vi "SetSendFileProperties.vi"(10 "acqusition timestamp":string, 11 "data group":string) -> (3 "send file properties":T1[](array[typedef]))   [LabVIEW 2017, in "FileManager.lvlib"]
uses:
  <vilib>/addons/InsightCM/Devices/Shared/Common/FileManager/FileManager.lvlib
  <vilib>/addons/InsightCM/MessageBus/Base/controls/KeyValuePair.ctl
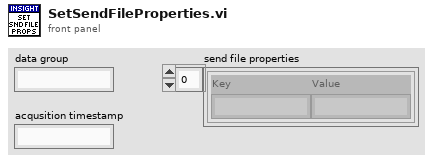
[diagram p1: front panel]
types:
  T1 = typedef "KeyValuePair.ctl" = cluster{"Key":string, "Value":string}
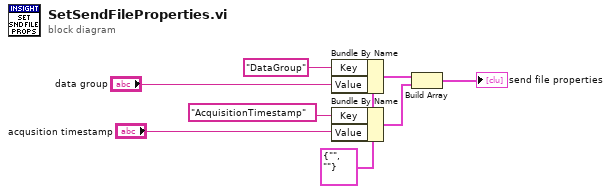
[diagram p0: block diagram]
diagram:
  w8 = T1 {"Key"="", "Value"=""} ("KeyValuePair")
  n1 = Bundle By Name(cluster=w8, "Key"="DataGroup", "Value"="data group") -> (w2:T1)
  n2 = Bundle By Name(cluster=w8, "Key"="AcquisitionTimestamp", "Value"="acqusition timestamp") -> (w6:T1)
  n3 = Build Array(w2, w6) -> (→"send file properties":T1[])
